vi "XY Graph Is Special Event.vi"(8 "Error In":errorcluster, 10 "XY Graph Event":T3) -> (0 "Error Out":errorcluster, 2 "XY Graph Event":T3, 3 "Special Event":bool)   [LabVIEW 2021, in "XY Graph Add-Ons.lvlib"]
uses:
  XY Graph Add-Ons.lvlib
  XY Graph Event.ctl
  <vilib>/Utility/miscctls.llb/LVPoint32TypeDef.ctl
  XY Graph Menu Items.ctl
panel:
  in  "Fit Models":T1(ring)
  in  "XY Graph Menu Items":T2=enum."Fit Menu"
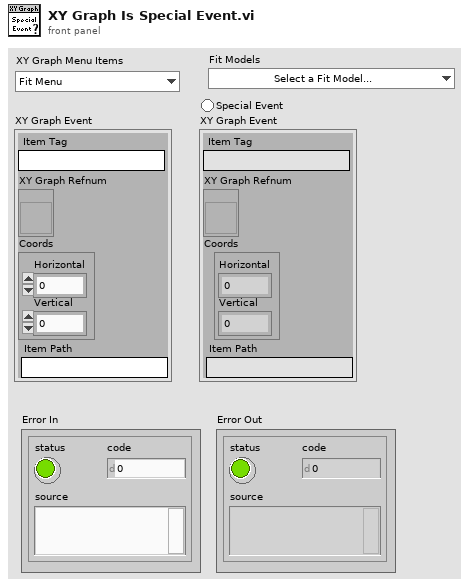
[diagram p1: front panel]
types:
  T1 = enum16{"Select a Fit Model...", "           Single Peak", "Gaussian", "Asymmetric Gaussian", "Lorentzian", "Asymmetric Lorentzian", "Gaussian/Lorentzian", "Lorentzian/Gaussian", "           Double Peak", "Two Gaussians", "Two Asymmetric Gaussians", "Two H-Connected Gaussians", "Two T-Connected Gaussians", "Two H-Connected Asymmetric Gaussians", "Two T-Connected Asymmetric Gaussians", "           Triple Peak", "Three Gaussians", "Three Asymmetric Gaussians", "              Decays", "Single Exponential", "Two Exponentials", "               ACF", "2D Gaussian ACF", "2D Gaussian + Blinking ACF", "2D Gaussian + Flow ACF", "3D Gaussian ACF", "3D Gaussian + Blinking ACF", "             Multiplot", "2D Gaussian ACF & 2D Gaussian + Flow ACF"}
  T2 = typedef "XY Graph Add-Ons.lvlib/XY Graph Menu Items.ctl" = enum16{"-", "Histogram", "Edit Plot", "Select Plots...", "Select All Plots", "Deselect Plots...", "Deselect All Plots", "Invert Plots Selection", "Set Style of Selected Plots", "Set Axes of Selected Plots", "Delete Plot", "Delete Selected Plots", "Clear Graph", "Save Plot", "Save Selected Plots", "Save All Plots", "Load Plot(s)", "Add Selected Plots", "Single Plot Arithmetic", "Fit Menu", "Copy Data", "Export Menu", "Visible Items Menu", "Show/Hide Grid", "Show/Hide Tool Panels"}
  T3 = typedef "XY Graph Add-Ons.lvlib/XY Graph Event.ctl" = cluster{"Item Tag":string, "XY Graph Refnum":refnum<vi>, "Coords":T4, "Item Path":string}
  T4 = typedef "LVPoint32TypeDef.ctl" = cluster{"Horizontal":i32, "Vertical":i32}
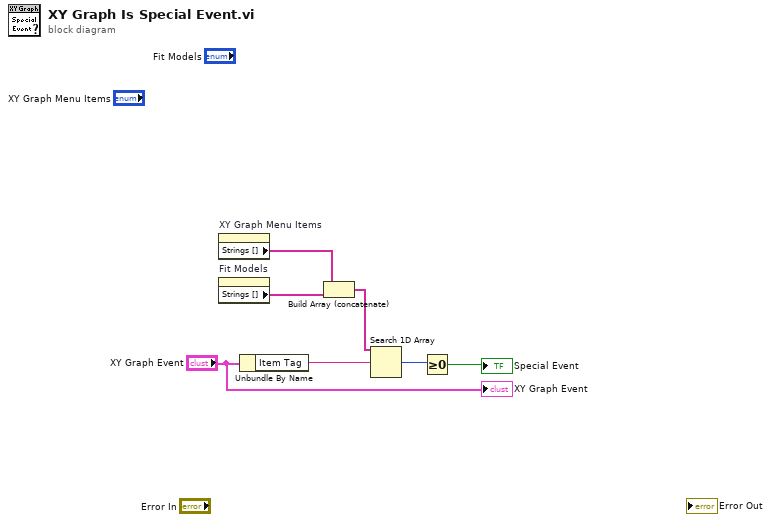
[diagram p0: block diagram]
diagram:
  n1 = property on="XY Graph Menu Items" class="Enum (strict)"() -> ("Strings []"=w2:string[])  [unwired: 2 in, 2 out]
  n2 = property on="Fit Models" class="Enum (strict)"() -> ("Strings []"=w1:string[])  [unwired: 2 in, 2 out]
  n3 = Unbundle By Name("XY Graph Event") -> ("Item Tag"=w7:string)
  n4 = Build Array (concatenate)(w2, w1) -> (w3:string[])
  n5 = Search 1D Array(1D array=w3, element=w7) -> (index of element=w6:i32)  [unwired: 1 in]
  n6 = Greater Or Equal To 0?(x=w6) -> (x >= 0?=→"Special Event":bool)
  "XY Graph Event" <- "XY Graph Event"
